vi "Gate-General Window.vi"(8 "window":T1 items=["Rectangle"=0, "Hanning"=1, "Hamming"=2, "Blackman-Harris"=3, "Exact Blackman"=4, "Blackman"=5, "Flat Top"=6, "4 Term B-Harris "=7, "7 Term B-Harris"=8, "Low Sidelobe"=9, "Blackman Nuttall"=11, "Triangle"=30, "Bartlett-Hanning"=31, "Bohman"=32, "Parzen"=33, "Welch"=34, "Kaiser"=60, "Dolph-Chebyshev"=61, "Gaussian"=62], 10 "Nramp":i32, 11 "X":dbl[](array[numeric])) -> (3 "X windowed":dbl[](array[numeric]))   [LabVIEW 2020]
uses:
  <vilib>/Analysis/4window.llb/windowTd.ctl
  <vilib>/Analysis/4window.llb/Symmetric Window (DBL).vi
  <vilib>/Analysis/NI_AALPro.lvlib
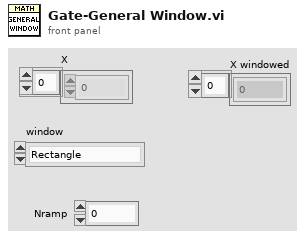
[diagram p1: front panel]
types:
  T1 = typedef "NI_AALPro.lvlib/windowTd.ctl" = u32
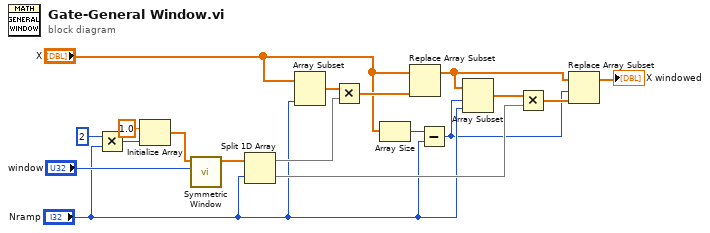
[diagram p0: block diagram]
diagram:
  n1 = Multiply(x=2 ("y"), y="Nramp") -> (x*y=w16:i32)
  n2 = Initialize Array(1.0 ("element"), w16) -> (w14:dbl[])
  n3 = call-poly <vilib>:"Symmetric Window.vi"("window"="window", "X"=w14) -> ("Windowed X"=w13:dbl[])  [unwired: 8 in, 1 out]
  n4 = Split 1D Array(array=w13, index="Nramp") -> (first subarray=w11:dbl[], second subarray=w6:dbl[])
  n5 = Array Subset(array="X", length="Nramp") -> (w12:dbl[])  [unwired: 1 in]
  n6 = Multiply(x=w12, y=w11) -> (x*y=w10:dbl[])
  n7 = Array Size(array="X") -> (size(s)=w4:i32)
  n8 = Replace Array Subset(array="X", new element=w10) -> (w7:dbl[])  [unwired: 1 in]
  n9 = Subtract(x=w4, y="Nramp") -> (x-y=w1:i32)
  n10 = Array Subset(array=w7, index=w1, length="Nramp") -> (w9:dbl[])
  n11 = Multiply(x=w9, y=w6) -> (x*y=w8:dbl[])
  n12 = Replace Array Subset(array=w7, new element=w8, index=w1) -> (→"X windowed":dbl[])
